vi "Set Position.vi"(8 "error in (no error)":errorcluster, 11 "Position":i32) -> (0 "error out":errorcluster)   [LabVIEW 2015]
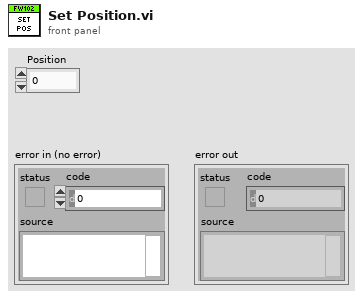
[diagram p1: front panel]
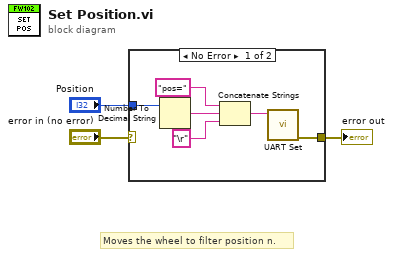
[diagram p0: block diagram]
diagram:
  # "Moves the wheel to filter position n."
  n1 = case shown="No Error" "error in (no error)" {
    selector: "error in (no error)" -> [_ w10]
    tunnel: [w9 w10] -> w3
    tunnel: "Position" -> [w8 _]
    frame No Error {
      n2 = Number To Decimal String(number=w8) -> (decimal integer string=w7:string)  [unwired: 1 in]
      n3 = Concatenate Strings("pos=" ("Input Command String"), w7, "\r" ("string")) -> (w4:string)
      n4 = call "UART Set.vi"("Command"=w4) -> ("error out"=w9:errorcluster)  [unwired: 10 in]
    }
    frame Error {
    }
  }
  "error out" <- w3
